vi "연속 읽기.vi"() -> ()   [LabVIEW 2014]
uses:
  <vilib>/Instr/_visa.llb/VISA Configure Serial Port (Instr).vi
panel:
  out "숫자형":i32=9
  out "에러 출력":errorcluster={"status"=FALSE, "code"=1073676294, "source"="XGB 통신.vi->연속 읽기.vi 안에 VISA 읽기"}
  in  "parity (0:none)":enum16{"None", "Odd", "Even", "Mark", "Space"}(ring) caption="패리티(0:없음)"
  in  "data bits (8)":u16=8 caption="데이터 비트(8)" min=5 max=8 step=1
  out "read buffer":string
  in  "baud rate (9600)":u32=115200 caption="보 전송속도(9600)"
  in  "VISA resource name":refnum<visa-resource-name>="COM1" caption="VISA 리소스 이름"
  in  "요구 프레임":string="\u000500RSB07%TW000032\u0004"
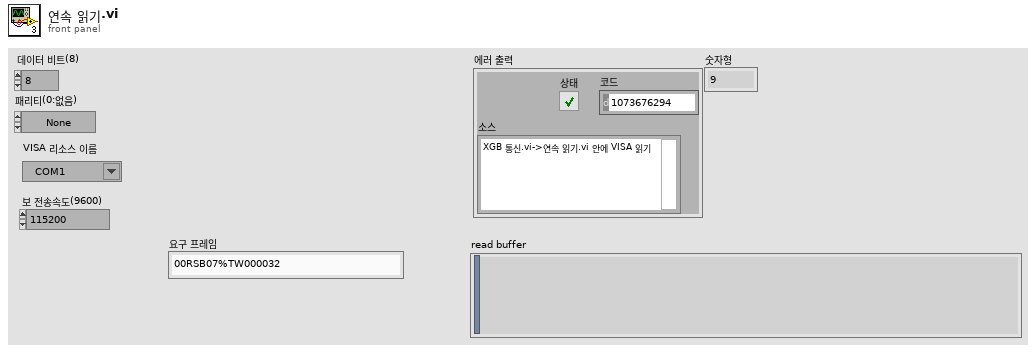
[diagram p1: front panel]
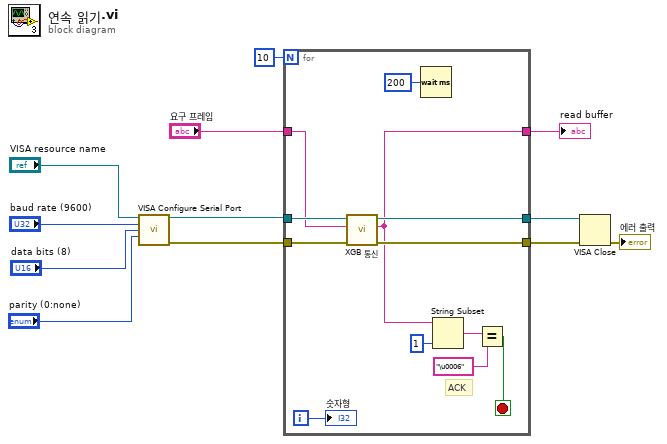
[diagram p0: block diagram]
diagram:
  n1 = call-poly "VISA Configure Serial Port"("VISA resource name"="VISA resource name", "baud rate (9600)"="baud rate (9600)", "data bits (8)"="data bits (8)", "parity (0:none)"="parity (0:none)") -> ("VISA resource name out"=w12:refnum<visa-resource-name>, "error out"=w10:errorcluster)  [unwired: 10 in]
  n2 = for {
    N: 10 -> [_]
    tunnel: w10 -> [w22]
    tunnel: [w21] -> w4
    tunnel: w12 -> [w24]
    tunnel: [w23] -> w11
    tunnel: "요구 프레임" -> [w20]
    tunnel: [w16] -> w2
    i -> [w13]
    stop <- w15 stop-if-true
    # "ACK"
    n3 = call "XGB 통신.vi"("error in (no error)"=w22, "String"=w20, "VISA Refnum in"=w24) -> ("error out"=w21:errorcluster, "read buffer"=w16:string, "VISA Refnum out"=w23:refnum<visa-resource-name>)  [unwired: 5 in, 1 out]
    n4 = Wait (ms)(milliseconds to wait=u32 200 ("대기 시간(ms)")) -> ()  [unwired: 1 out]
    n5 = String Subset(string=w16, length (rest)=1 ("length (rest)")) -> (substring=w18:string)  [unwired: 1 in]
    n6 = Equal?(x=w18, y="\u0006") -> (x = y?=w15:bool)
    "숫자형" <- w13
  }
  "read buffer" <- w2
  n7 = VISA Close(VISA resource name=w11, error in (no error)=w4) -> (error out=→"에러 출력":errorcluster)
